vi "niDTS BT BDR Rx Test Get Documentation.vi"(0 "RX Test Handle In":T1, 11 "error in (no error)":errorcluster) -> (4 "RX Test Handle Out":T1, 8 "Documentation":T2, 15 "error out":errorcluster)   [LabVIEW 2014, in "niDTS BT.lvlib"]
uses:
  niDTS BT.lvlib
  Framework/Test/Includes/niDTS Test INC Documentation.ctl
  BDR Tx Test/Includes/niDTS BT Rx Test INC Handle.ctl
  Rx Test/Objects/BASE_class/niDTS BT Rx Test.lvclass
  Framework/niDTS Framework.lvlib
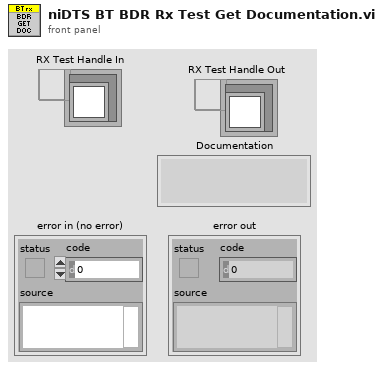
[diagram p1: front panel]
types:
  T1 = typedef "niDTS BT.lvlib/niDTS BT Rx Test INC Handle.ctl" = refnum<data-value>
  T2 = typedef "niDTS Framework.lvlib/niDTS Test INC Documentation.ctl" = string
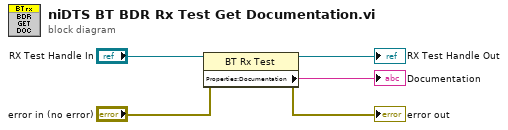
[diagram p0: block diagram]
diagram:
  n1 = property class="BT Rx Test"(reference="RX Test Handle In", error in="error in (no error)") -> (reference out=→"RX Test Handle Out":T1, error out=→"error out":errorcluster, "Properties:Documentation"=→"Documentation":T2)
